vi "set ciphers.vi"(8 "error in":errorcluster, 10 "ciphers":string, 11 "lvlibretls configurable context in":refnum<class "lvlibretls configurable context.lvclass">) -> (0 "error out":errorcluster, 3 "lvlibretls configurable context out":refnum<class "lvlibretls configurable context.lvclass">)   [LabVIEW 2016, in "lvlibretls configurable context.lvclass"]
doc: "tls_config_set_ciphers() sets the list of ciphers that may be used. Lists of ciphers are specified by name, and the permitted names are:\n\nsecure (or alias default)\ncompat\nlegacy\ninsecure (or alias all)\n\nAlternatively, libssl cipher strings can be specified. See the CIPHERS section of openssl(1) for further information, below:\n\nDEFAULT\nThe default cipher list. This is determined at compile time and is currently ALL:!aNULL:!eNULL:!SSLv2. This must be the first cipher string specified.\n \nCOMPLEMENTOFDEFAULT\nThe ciphers included in ALL, but not enabled by default. Currently this is ADH. Note that this rule does not cover eNULL, which is not included by ALL (use COMPLEMENTOFALL if necessary).\n \nALL\nAll cipher suites except the eNULL ciphers, which must be explicitly enabled.\n \nCOMPLEMENTOFALL\nThe cipher suites not enabled by ALL, currently being eNULL.\n \nHIGH\n“High” encryption cipher suites. This currently means those with key lengths larger than 128 bits.\n \nMEDIUM\n“Medium” encryption cipher suites, currently those using 128-bit encryption.\n \nLOW\n“Low” encryption cipher suites, currently those using 64- or 56-bit encryption algorithms.\n \n \neNULL, NULL\nThe “NULL” ciphers; that is, those offering no encryption. Because these offer no encryption at all and are a security risk, they are disabled unless explicitly included.\n \n \naNULL\nThe cipher suites offering no authentication. This is currently the anonymous DH algorithms. These cipher suites are vulnerable to a “man in the middle” attack, so their use is normally discouraged.\n \n \nkRSA, RSA\nCipher suites using RSA key exchange.\n \n \nkEDH\nCipher suites using ephemeral DH key agreement.\n \n \naRSA\nCipher suites using RSA authentication, i.e. the certificates carry RSA keys.\n \n \naDSS, DSS\nCipher suites using DSS authentication, i.e. the certificates carry DSS keys.\n \n \nTLSv1\nTLS v1.0 cipher suites.\n \n \nDH\nCipher suites using DH, including anonymous DH.\n \n \nADH\nAnonymous DH cipher suites.\n \n \nAES\nCipher suites using AES.\n \n \n3DES\nCipher suites using triple DES.\n \n \nDES\nCipher suites using DES (not triple DES).\n \n \nRC4\nCipher suites using RC4.\n \n \nCAMELLIA\nCipher suites using Camellia.\n \n \nCHACHA20\nCipher suites using ChaCha20.\n \n \nIDEA\nCipher suites using IDEA.\n \n \nMD5\nCipher suites using MD5.\n \n \nSHA1, SHA\nCipher suites using SHA1."
uses:
  lvlibretls configurable context.lvclass
  lvlibretls configurable context.lvclass/lvlibretls configurable context.ctl
  lv tls dll.lvlib
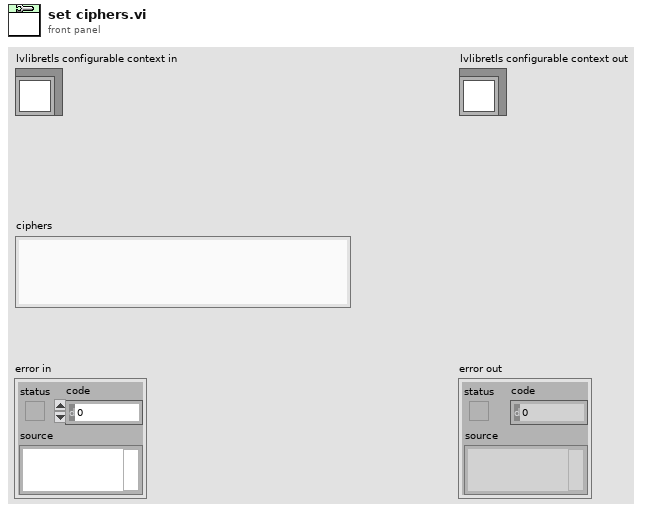
[diagram p1: front panel]
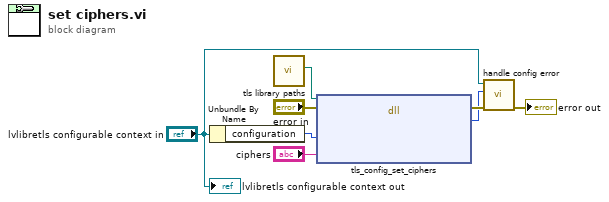
[diagram p0: block diagram]
diagram:
  n1 = Unbundle By Name("lvlibretls configurable context in") -> ("configuration"=w7:u64)
  n2 = call "tls library paths.vi"() -> ("libtls"=w8:path)  [unwired: 8 in, 3 out]
  n3 = dll-call lib="C:/Users/IEUser/Desktop/tlssimple/libtls-15.dll" fn="tls_config_set_ciphers"(path in=w8, error in="error in", "config"=w7, "ciphers"="ciphers") -> (error out=w6:errorcluster, "return"=w5:i32)  [unwired: 3 in, 1 out]
  n4 = call "handle config error.vi"("error in"=w6, "return"=w5, "lvlibretls configurable context in"="lvlibretls configurable context in") -> ("error out"=→"error out":errorcluster)  [unwired: 8 in]
  "lvlibretls configurable context out" <- "lvlibretls configurable context in"
